vi "MelFilterBank.vi"(6 "No of filters":i32=36, 8 "MaxFreq":dbl=5400.0, 9 "MinFreq":dbl=130.0) -> (2 "Triangle Pattern":dbl[][](array[numeric]))   [LabVIEW 2013]
uses:
  <vilib>/Analysis/1siggen.llb/General Aperiodic Triangle.vi
  <vilib>/Analysis/NI_AALBase.lvlib
panel:
  out "Triangle filters":dbl[][](graph)
  out "Centre frequencies":dbl[](array[numeric])
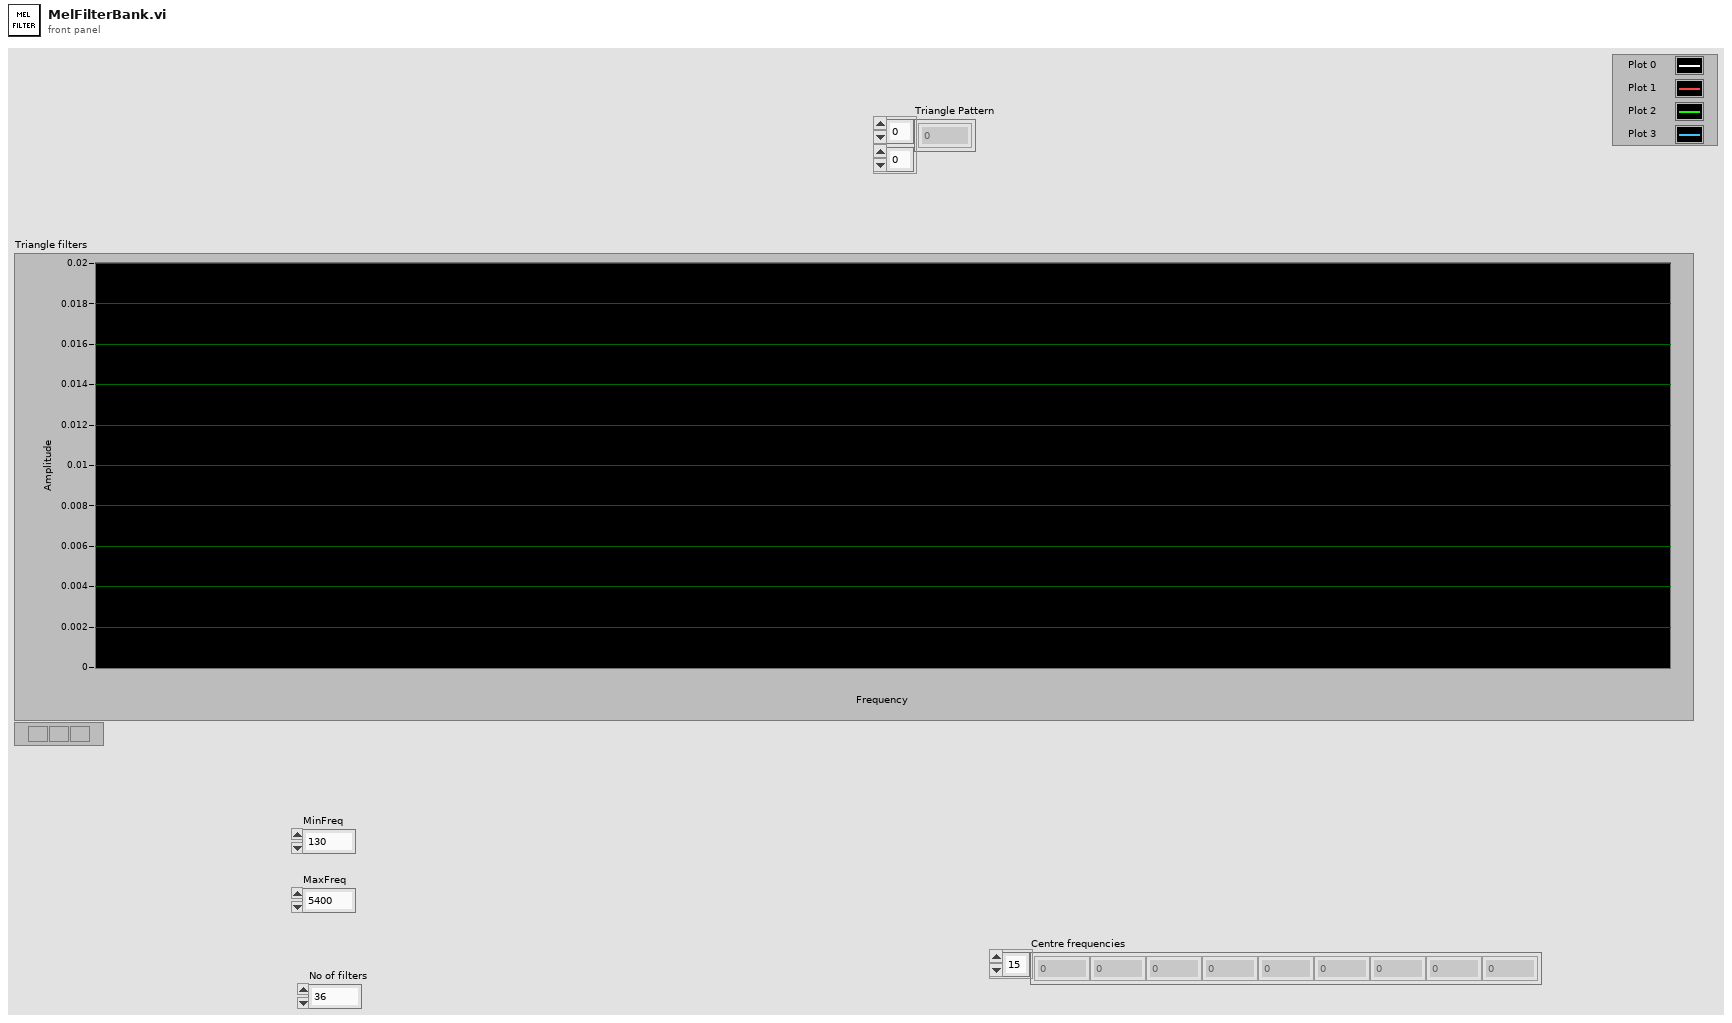
[diagram p1: front panel]
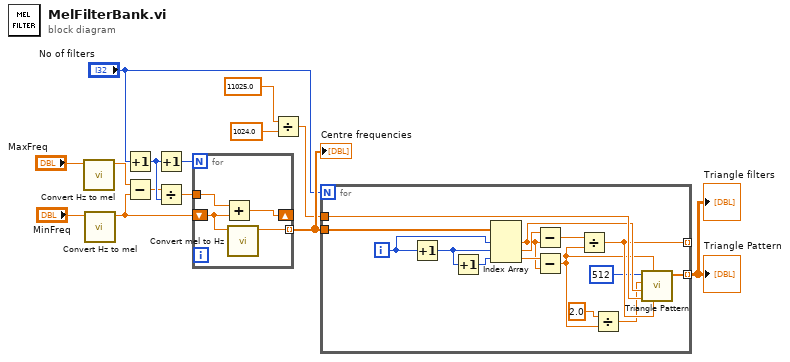
[diagram p0: block diagram]
diagram:
  n1 = call "Convert Hz to mel.vi"("Hz"="MaxFreq") -> ("mel"=w3:dbl)  [unwired: 10 in]
  n2 = call "Convert Hz to mel.vi"("Hz"="MinFreq") -> ("mel"=w6:dbl)  [unwired: 10 in]
  n3 = Increment(x="No of filters") -> (x+1=w7:i32)
  n4 = Subtract(x=w3, y=w6) -> (x-y=w4:dbl)
  n5 = Increment(x=w7) -> (x+1=w2:i32)
  n6 = Divide(x=w4, y=w7) -> (x/y=w5:dbl)
  n7 = for {
    N: w2 -> [_]
    tunnel: w5 -> [w16]
    tunnel: [w18] -> w12 mode=indexing
    shift-right: [w15] -> _
    shift-left: w6 -> [w17]
    n8 = Add(x=w16, y=w17) -> (x+y=w15:dbl)
    n9 = call "Convert mel to Hz.vi"("mel"=w17) -> ("Hz"=w18:dbl)  [unwired: 10 in]
  }
  "Centre frequencies" <- w12
  n10 = Divide(x=11025.0, y=1024.0) -> (x/y=w10:dbl)
  n11 = for {
    N: "No of filters" -> [_]
    tunnel: [w30] -> w11 mode=indexing
    tunnel: w12 -> [w29]
    tunnel: w10 -> [w28]
    tunnel: [w23] -> _ mode=indexing
    i -> [w33]
    n12 = Increment(x=w33) -> (x+1=w32:i32)
    n13 = Increment(x=w32) -> (x+1=w31:i32)
    n14 = Index Array(array=w29, index #1=w33, index #2=w32, index #3=w31) -> (element #1=w25:dbl, element #2=w26:dbl, element #3=w27:dbl)
    n15 = Subtract(x=w26, y=w25) -> (x-y=w24:dbl)
    n16 = Subtract(x=w27, y=w25) -> (x-y=w22:dbl)
    n17 = Divide(x=w24, y=w22) -> (x/y=w23:dbl)
    n18 = Divide(x=2.0, y=w22) -> (x/y=w20:dbl)
    n19 = call <vilib>:"Triangle Pattern.vi"("asymmetry"=w23, "width (s)"=w22, "delta t (s)"=w28, "delay (s)"=w25, "amplitude"=w20, "samples"=512) -> ("Triangle Pattern"=w30:dbl[])  [unwired: 4 in, 1 out]
  }
  "Triangle filters" <- w11
  "Triangle Pattern" <- w11
